vi "Configure Arm Layer Trigger Source.vi"(6 "Arm Timer Interval (0.1 s)":dbl=0.1, 8 "error in (no error)":errorcluster, 9 "Arm Count (1)":i32=1, 10 "Arm Source (1: Immediate)":i32(ring)=1 items=["Hold", "Immediate", "Real-time Clock", "Manual", "Bus", "Trigger Link", "External Triggering", "Timer", "STest", "PSTest", "NSTest", "BSTest"], 11 "VISA resource name":refnum<visa-resource-name>) -> (0 "error out":errorcluster, 3 "VISA resource name out":refnum<visa-resource-name>)   [LabVIEW 2020, in "Keithley 6517.lvlib"]
doc: "Configures the count and source for the Arm Layer (Arm1) of the trigger model. \n\n<B>Note:</B>\n(1)<B>Models 6517A, 6517B:</B> The trigger model consists of 3 layers, the Arm Layer, the Scan Layer (Arm2), and the Measure Layer (Trigger).\n(2)<B>Model 6514:</B> The trigger model consists of 2 layers: Arm Layer & Measure Layer (Trigger)."
uses:
  <instrlib>/Keithley 6517/Keithley 6517.lvlib
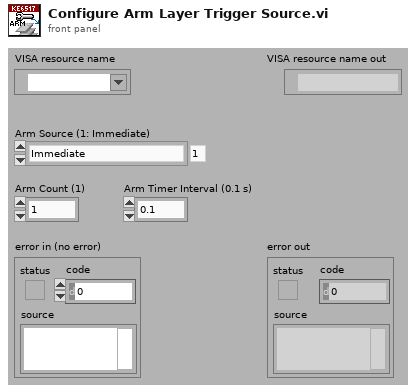
[diagram p1: front panel]
types:
  T1 = typedef "Keithley 6517.lvlib/Extended User Data.ctl" = cluster{"Instrument Model":i32}
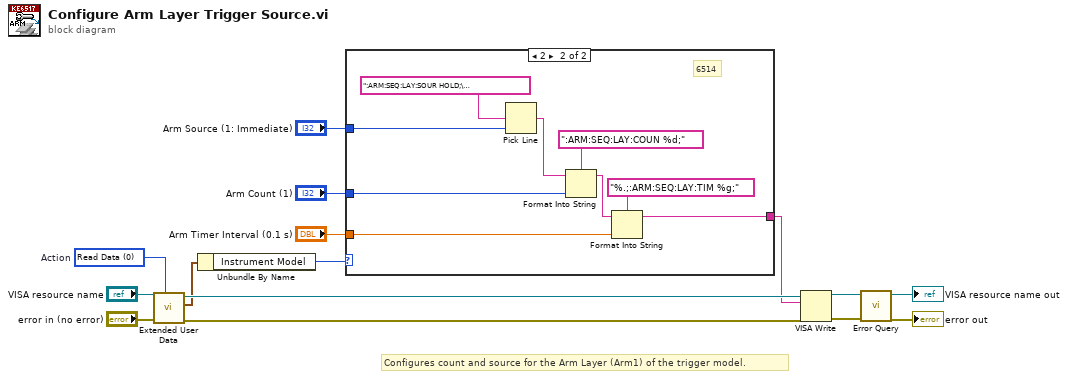
[diagram p0: block diagram]
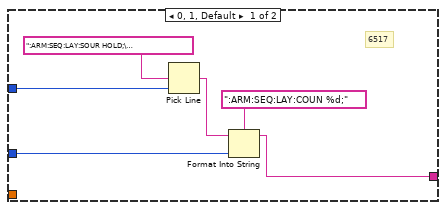
[diagram p2: hidden frame]
diagram:
  w3 = u16 0 items=["Read Data", "Write Data", "Clear Data", "Clear ALL Data"]  # Action
  # "Configures count and source for the Arm Layer (Arm1) of the trigger model."
  n1 = call <instrlib>:"Extended User Data.vi"("Action (0: Read Data)"=w3, "error in (no error)"="error in (no error)", "VISA resource name"="VISA resource name") -> ("error out"=w7:errorcluster, "User Data Out"=w5:T1, "VISA resource name out"=w6:refnum<visa-resource-name>)  [unwired: 6 in]
  n2 = Unbundle By Name(w5) -> ("Instrument Model"=w4:i32)
  n3 = case shown="2" w4 {
    tunnel: "Arm Count (1)" -> [w20 w29]
    tunnel: "Arm Source (1: Immediate)" -> [w19 w28]
    tunnel: "Arm Timer Interval (0.1 s)" -> [_ w23]
    tunnel: [w16 w22] -> w1
    frame 0, 1, Default {
      # "6517"
      n4 = Pick Line(multi-line string=":ARM:SEQ:LAY:SOUR HOLD;\n:ARM:SEQ:LAY:SOUR IMM;\n:ARM:SEQ:LAY:SOUR RTCL;\n:ARM:SEQ:LAY:SOUR MAN;\n:ARM:SEQ:LAY:SOUR BUS;\n:ARM:SEQ:LAY:SOUR TLIN;\n:ARM:SEQ:LAY:SOUR EXT;", line index=w19) -> (output string=w17:string)  [unwired: 1 in]
      n5 = Format Into String(format string=":ARM:SEQ:LAY:COUN %d;", initial string=w17, w20) -> (resulting string=w16:string)  [unwired: 1 in, 1 out]
    }
    frame 2 {
      # "6514"
      n6 = Pick Line(multi-line string=":ARM:SEQ:LAY:SOUR HOLD;\n:ARM:SEQ:LAY:SOUR IMM;\n:ARM:SEQ:LAY:SOUR RTCL;\n:ARM:SEQ:LAY:SOUR MAN;\n:ARM:SEQ:LAY:SOUR BUS;\n:ARM:SEQ:LAY:SOUR TLIN;\n:ARM:SEQ:LAY:SOUR EXT;\n:ARM:SEQ:LAY:SOUR TIM;\n:ARM:SEQ:LAY:SOUR STES;\n:ARM:SEQ:LAY:SOUR PST;\n:ARM:SEQ:LAY:SOUR NST;\n:ARM:SEQ:LAY:SOUR BST;\n\n\n\n", line index=w28) -> (output string=w26:string)  [unwired: 1 in]
      n7 = Format Into String(format string=":ARM:SEQ:LAY:COUN %d;", initial string=w26, w29) -> (resulting string=w24:string)  [unwired: 1 in, 1 out]
      n8 = Format Into String(format string="%.;:ARM:SEQ:LAY:TIM %g;", initial string=w24, w23) -> (resulting string=w22:string)  [unwired: 1 in, 1 out]
    }
  }
  n9 = VISA Write(VISA resource name=w6, write buffer=w1, error in (no error)=w7) -> (VISA resource name out=w14:refnum<visa-resource-name>, error out=w13:errorcluster)  [unwired: 1 out]
  n10 = call <instrlib>:"Error Query.vi"("error in (no error)"=w13, "VISA resource name"=w14) -> ("error out"=→"error out":errorcluster, "VISA resource name out"=→"VISA resource name out":refnum<visa-resource-name>)  [unwired: 6 in, 2 out]
